vi "LVIS_CustomError.vi"(8 "error in (no error)":errorcluster, 10 "Addiitional Info":string, 11 "Code":i32) -> (0 "error out":errorcluster)   [LabVIEW 2015]
doc: "Performs a lookup of the custom error code and appends any additional information to the error."
uses:
  Globals/LVIS_IsGlobal.vi
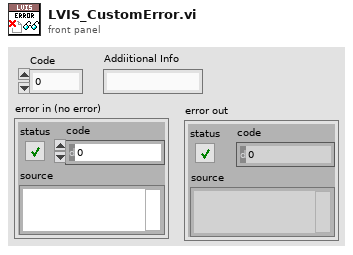
[diagram p1: front panel]
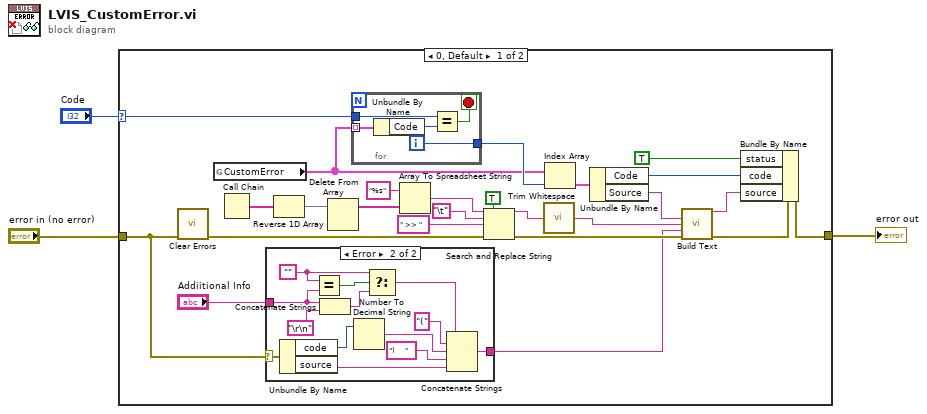
[diagram p0: block diagram]
diagram:
  n1 = case shown="0, Default" "Code" {
    selector: "Code" -> [w27 _]
    tunnel: "error in (no error)" -> [w10 w48]
    tunnel: [w12 w48] -> w3
    frame 0, Default {
      n2 = call <vilib>:"Clear Errors.vi"("error in (no error)"=w10) -> ("error out"=w11:errorcluster)  [unwired: 5 in, 1 out]
      n3 = global read "LVIS_IsGlobal.vi" "CustomError"() -> (w4:cluster{"Code":i32, "Source":string}[])
      n4 = Call Chain() -> (call chain=w18:string[])
      n5 = case shown="Error" w10 {
        selector: w10 -> [_ w41]
        tunnel: [w29 w42] -> w9
        tunnel: "Addiitional Info" -> [w29 w33]
        frame No Error {
        }
        frame Error {
          w30 = ""
          n6 = Unbundle By Name(w41) -> ("code"=w40:i32, "source"=w36:string)
          n7 = Equal?(x=w30, y=w33) -> (x = y?=w35:bool)
          n8 = Concatenate Strings(w33, "\r\n") -> (w34:string)
          n9 = Number To Decimal String(number=w40) -> (decimal integer string=w38:string)  [unwired: 1 in]
          n10 = Select(t=w30, s=w35, f=w34) -> (s? t:f=w31:string)
          n11 = Concatenate Strings(w31, "(", w38, ")     ", w36) -> (w42:string)
        }
      }
      n12 = Reverse 1D Array(array=w18) -> (reversed array=w17:string[])
      n13 = Delete From Array(array=w17) -> (array with subset deleted=w16:string[])  [unwired: 2 in, 1 out]
      n14 = for {
        tunnel: w4 -> [w47] mode=indexing
        tunnel: w27 -> [w44]
        tunnel: [w43] -> w26
        i -> [w43]
        stop <- w45 stop-if-true
        n15 = Unbundle By Name(w47) -> ("Code"=w46:i32)
        n16 = Equal?(x=w44, y=w46) -> (x = y?=w45:bool)
      }
      n17 = Array To Spreadsheet String(array=w16, 3:"%s" ("format string")) -> (spreadsheet string=w22:string)  [unwired: 1 in]
      n18 = Search and Replace String(replace all?=TRUE ("replace all? (F)"), input string=w22, search string="\t", replace string=" >> ", error in=w11) -> (result string=w15:string, error out=w23:errorcluster)  [unwired: 3 in, 2 out]
      n19 = call <vilib>:"Trim Whitespace.vi"("string"=w15) -> ("trimmed string"=w5:string)  [unwired: 1 in]
      n20 = Index Array(array=w4, index=w26) -> (element=w28:cluster{"Code":i32, "Source":string})
      n21 = Unbundle By Name(w28) -> ("Code"=w13:i32, "Source"=w6:string)
      n22 = call "Build Text"("Msg"=w6, "Source"=w5, "Info"=w9, "error in (no error)"=w23) -> ("Result"=w7:string, "error out"=w14:errorcluster)  [unwired: 10 in]
      n23 = Bundle By Name(cluster=w14, "status"=TRUE, "code"=w13, "source"=w7) -> (w12:errorcluster)
    }
    frame -1 {
    }
  }
  "error out" <- w3
